vi "LEP_RV_CreateOpBox.vi"(8 "error in (no error)":errorcluster, 11 "Title":string="µVision") -> (0 "error out":errorcluster)   [LabVIEW 2011]
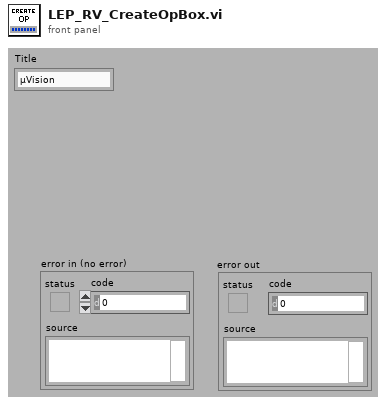
[diagram p1: front panel]
types:
  T1 = enum32{"Invalid", "Standard", "Closed", "Hidden", "Minimized", "Maximized"}
  T2 = enum32{"Bad", "Idle", "Run top level", "Running"}
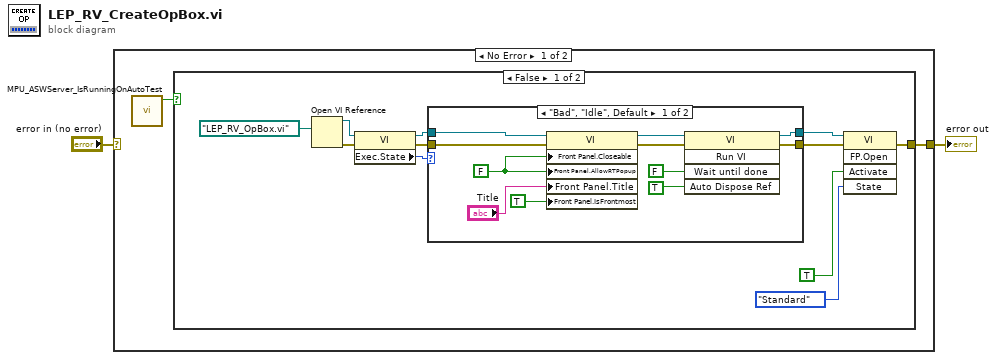
[diagram p0: block diagram]
diagram:
  n1 = case shown="No Error" "error in (no error)" {
    selector: "error in (no error)" -> [_ w29]
    tunnel: [w4 w29] -> w1
    frame No Error {
      n2 = call <vilib>:"MPU_ASWServer_IsRunningOnAutoTest.vi"() -> ("running in autotest?"=w3:bool)  [unwired: 1 in, 10 out]
      n3 = case shown="False" w3 {
        tunnel: [w5 _] -> w4
        frame False {
          n4 = Open VI Reference(vi path=path "LEP_RV_OpBox.vi") -> (vi reference=w11:refnum<vi>, error out=w14:errorcluster)  [unwired: 5 in]
          n5 = property class="VI"(reference=w11, error in=w14) -> (reference out=w6:refnum<vi>, error out=w13:errorcluster, "Exec.State"=w12:T2)
          n6 = case shown="\"Bad\", \"Idle\", Default" w12 {
            tunnel: [w23 w28] -> w8
            tunnel: w13 -> [w21 w28]
            tunnel: w6 -> [w22 w27]
            tunnel: [w24 w27] -> w7
            frame "Bad", "Idle", Default {
              w20 = FALSE ("Front Panel Window:Closeable")
              n7 = property class="VI"(reference=w22, error in=w21, "Front Panel.Closeable"=w20, "Front Panel.AllowRTPopup"=w20, "Front Panel.Title"="Title", "Front Panel.IsFrontmost"=TRUE ("Front Panel Window:Is Frontmost")) -> (reference out=w17:refnum<vi>, error out=w16:errorcluster)
              n8 = invoke class="VI" method="Run VI"(reference=w17, error in=w16, "Wait until done"=FALSE ("Wait Until Done"), "Auto Dispose Ref"=TRUE ("Auto Dispose Reference")) -> (reference out=w24:refnum<vi>, error out=w23:errorcluster)  [unwired: 1 in, 3 out]
            }
            frame "Run top level", "Running" {
            }
          }
          n9 = invoke class="VI" method="FP.Open"(reference=w7, error in=w8, "Activate"=TRUE ("Activate?"), "State"=T1."Standard") -> (error out=w5:errorcluster)  [unwired: 1 in, 4 out]
        }
        frame True {
          # "We do not want any pop up dialogues if we are running an auto test."
        }
      }
    }
    frame Error {
    }
  }
  "error out" <- w1
